vi "AcquisitionDataCSV.vi"() -> ()   [LabVIEW 2016]
uses:
  <vilib>/MakerHub/LINX/Public/Utilities/Open Serial.vi
  <vilib>/Utility/file.llb/Write Delimited Spreadsheet (DBL).vi
  <vilib>/MakerHub/LINX/LMH-LINX.lvlib
panel:
  out "Input":dbl(graph)
  out "Velocity (RPM)":dbl(graph)
  out "Position (Degrees)":dbl(graph)
  in  "T":u32
  out "Loop Rate (Hz)":u32
  in  "Number Of Pulses":i32
  in  "Source Voltage":dbl
  in  "Voltage":dbl
  in  "IN 4":u8
  in  "IN3":u8
  in  "PWM Channel":u8
  in  "stop":bool
  in  "Serial Port":refnum<visa-resource-name>="N/A"
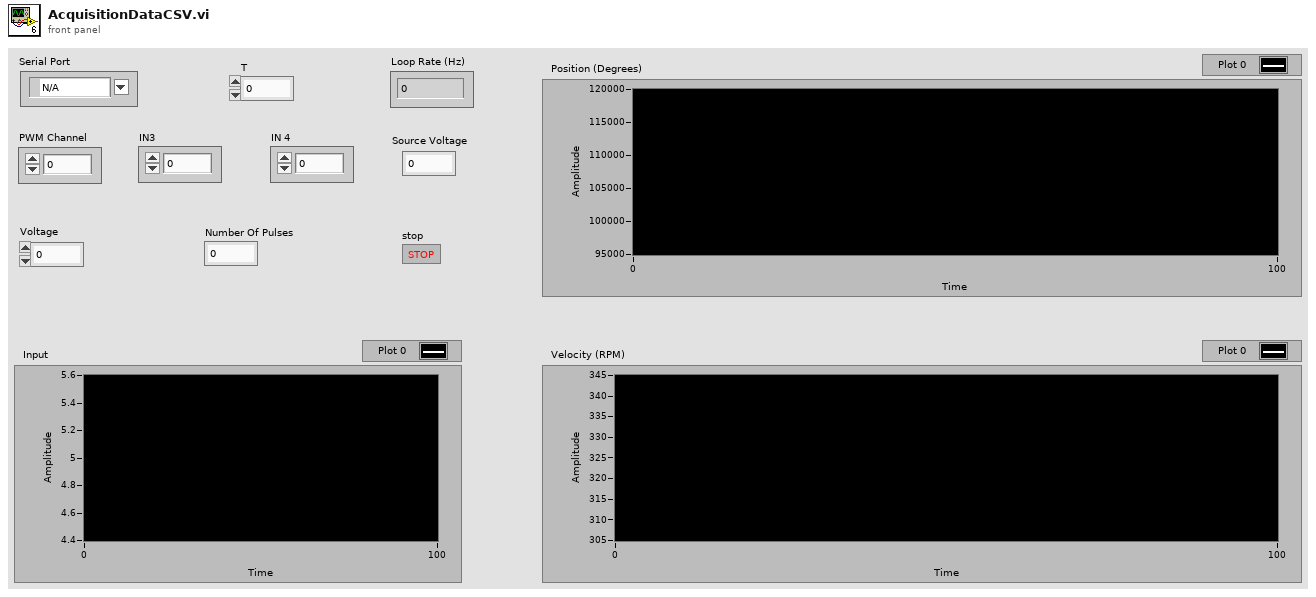
[diagram p1: front panel]
types:
  T1 = typedef "LMH-LINX.lvlib/LINX Ref.ctl" = cluster{"IO":T2, "Interface":T3, "LINX Device Config":T4}
  T2 = typedef "LMH-LINX.lvlib/Platform.ctl" = enum16{"Remote", "Local"}
  T3 = typedef "LMH-LINX.lvlib/Interface.ctl" = enum16{"Serial", "TCP"}
  T4 = typedef "LMH-LINX.lvlib/Device.lvlib/LINX Device Config.ctl" = cluster{"Interface":T3, "COM Port":refnum<visa-resource-name>, "TCP Configuration":T5, "Device Family":u8, "Device ID":u8, "Device Name":string, "TCP Ref":refnum<k5>, "Channels":T6}
  T5 = typedef "LMH-LINX.lvlib/Device.lvlib/TCP Config.ctl" = cluster{"IP Address":string, "Port":u16}
  T6 = typedef "LMH-LINX.lvlib/Channels.ctl" = cluster{"DI":u8[], "DO":u8[], "AI":u8[], "AO":u8[], "PWM":u8[], "QE":u8[], "UART":u8[], "I2C 2":u8[], "SPI":u8[], "CAN":u8[], "Servo":u8[], "AI Ref (V)":dbl, "AI Resolution (Bits)":u8, "AO Ref (V)":dbl, "AO Resolution (Bits)":u8}
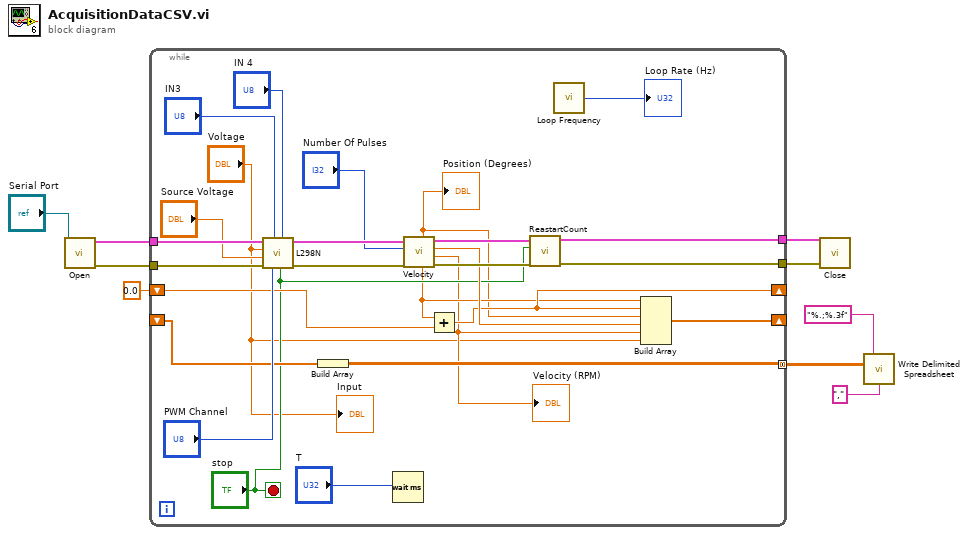
[diagram p0: block diagram]
diagram:
  n1 = call-poly <vilib>:"Open.vi"("Serial Port"="Serial Port") -> ("Error Out"=w5:errorcluster, "LINX Resource"=w6:T1)  [unwired: 8 in, 1 out]
  n2 = while {
    tunnel: w6 -> [w32]
    tunnel: w5 -> [w31]
    shift-right: [w15] -> _
    shift-left: 0.0 ("dt") -> [w26]
    tunnel: [w23] -> w4
    tunnel: [w22] -> w3
    shift-right: [w19] -> _
    shift-left: _ -> [w18]
    tunnel: [w17] -> w1 mode=concatenating
    stop <- "stop" stop-if-true
    n3 = call "L298N.vi"("Turn Off"="stop", "IN 4"="IN 4", "PWM Channel"="PWM Channel", "IN3"="IN3", "Error In"=w31, "Source Voltage"="Source Voltage", "Voltage"="Voltage", "LINX Resource IN"=w32) -> ("Error Out"=w28:errorcluster, "LINX Resource OUT"=w29:T1)  [unwired: 2 in]
    n4 = Build Array(w18) -> (w17:dbl[][])
    n5 = Wait (ms)(milliseconds to wait="T") -> ()  [unwired: 1 out]
    n6 = call "Velocity.vi"("Error In"=w28, "Number of pulses"="Number Of Pulses", "LINX Resource IN"=w29) -> ("Error Out"=w24:errorcluster, "RPM"=w11:dbl, "Velocity (Degrees/Seconds)"=w21:dbl, "LINX Resource OUT"=w25:T1, "dt"=w14:dbl, "Position (Degrees)"=w12:dbl)  [unwired: 3 in]
    "Position (Degrees)" <- w12
    "Velocity (RPM)" <- w11
    n7 = Add(x=w14, y=w26) -> (x+y=w15:dbl)
    n8 = call "ReastartCount.vi"("Error In"=w24, "Activate"="stop", "LINX Resource IN"=w25) -> ("Error Out"=w22:errorcluster, "LINX Resource OUT"=w23:T1)  [unwired: 7 in]
    n9 = call <vilib>:"Loop Frequency.vi"() -> ("Loop Rate (Hz)"=→"Loop Rate (Hz)":u32)
    n10 = Build Array(w14, w15, w12, w21, w11, "Voltage") -> (w19:dbl[])
    "Input" <- "Voltage"
  }
  n11 = call <vilib>:"Close.vi"("Error In"=w3, "LINX Resource"=w4) -> ()  [unwired: 9 in, 1 out]
  n12 = call-poly <vilib>:"Write Delimited Spreadsheet.vi"("format (%.3f)"="%.;%.3f", "2D data"=w1, "delimiter (\\t)"="," ("delimiter (\\t)")) -> ()  [unwired: 11 in, 2 out]
